vi "Update Rate.vi"(8 "error in (no error)":errorcluster, 11 "Model in":refnum<class "Model.lvclass">) -> (0 "error out":errorcluster, 3 "Model out":refnum<class "Model.lvclass">)   [LabVIEW 2015, in "Model.lvclass"]
uses:
  Model.lvclass
  Model.lvclass/Model.ctl
  <userlib>/Common/ILC/ILC/ILC.lvclass/ILC.ctl
  <userlib>/Common/ILC/ILC/ILC.lvclass
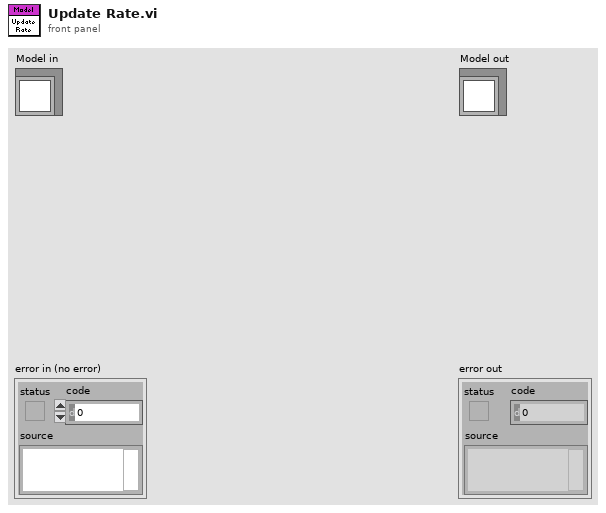
[diagram p1: front panel]
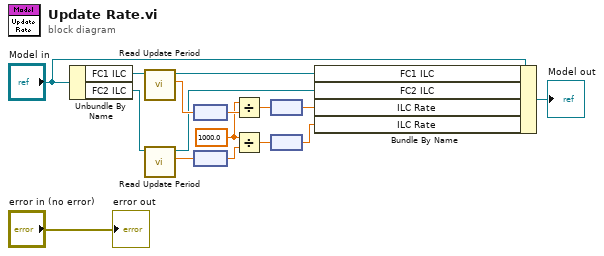
[diagram p0: block diagram]
diagram:
  w5 = 1000.0 ("x")
  n1 = Unbundle By Name("Model in") -> ("FC1 ILC"=w14:refnum<class "ILC.lvclass">, "FC2 ILC"=w15:refnum<class "ILC.lvclass">)
  n2 = call <userlib>:"Read Update Period.vi"("ILC in"=w14) -> ("Update Period"=w8:dbl[unit], "ILC out"=w7:refnum<class "ILC.lvclass">)  [unwired: 9 in]
  n3 = call <userlib>:"Read Update Period.vi"("ILC in"=w15) -> ("Update Period"=w11:dbl[unit], "ILC out"=w6:refnum<class "ILC.lvclass">)  [unwired: 9 in]
  n4 = node(w8) -> (w9:dbl)
  n5 = node(w11) -> (w10:dbl)
  n6 = Divide(x=w5, y=w9) -> (x/y=w4:dbl)
  n7 = Divide(x=w5, y=w10) -> (x/y=w2:dbl)
  n8 = node(w4) -> (w3:dbl[unit])
  n9 = node(w2) -> (w1:dbl[unit])
  n10 = Bundle By Name(cluster="Model in", "FC1 ILC"=w7, "FC2 ILC"=w6, "ILC Rate"=w3, "ILC Rate"=w1) -> (→"Model out":refnum<class "Model.lvclass">)
  "error out" <- "error in (no error)"
